vi "WPI_I2CBusCache.vi"(7 "Operation":T2, 8 "error in":errorcluster, 9 "I2C Bus":T1, 11 "Device Address":u8) -> (0 "error out":errorcluster, 2 "Allocated?":bool, 3 "Device Address Allocated":u8)   [LabVIEW 2017]
doc: "This software is licensed. Open the labview\\readme\\WPI Robotics Library Open Source License.txt file for more information."
uses:
  <vilib>/Rock Robotics/WPI/SPI/WPI_SPIBusCacheOp.ctl
  <vilib>/Rock Robotics/SystemInterfaces/i2clib/i2c_bus.ctl
  <vilib>/Rock Robotics/WPI/PWM/WPI_PWMChannelCacheOp.ctl
  <vilib>/Rock Robotics/WPI/MXP/WPI_MXP I2C Bus to first MXP Pin.vi
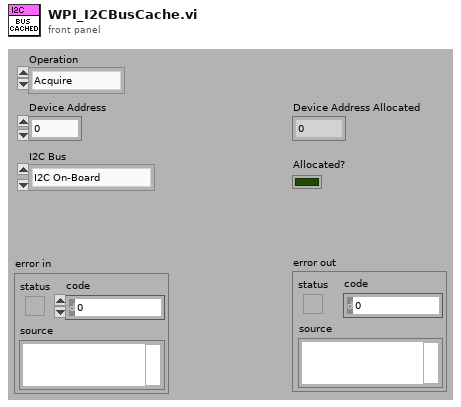
[diagram p1: front panel]
types:
  T1 = typedef "i2c_bus.ctl" = enum16{"I2C On-Board", "I2C MXP", "Invalid"}
  T2 = typedef "WPI_SPIBusCacheOp.ctl" = enum16{"Acquire", "Release", "Status"}
  T3 = typedef "WPI_PWMChannelCacheOp.ctl" = enum16{"Acquire", "Release", "Status"}
  T4 = typedef "WPI_MXP Shared MXP Pin.ctl" = enum16{"11", "13", "15", "17", "19", "21", "23", "25", "27", "29", "31", "18", "22", "26", "32", "34", "Invalid"}
  T5 = typedef "Semaphore RefNum" = refnum<k1>
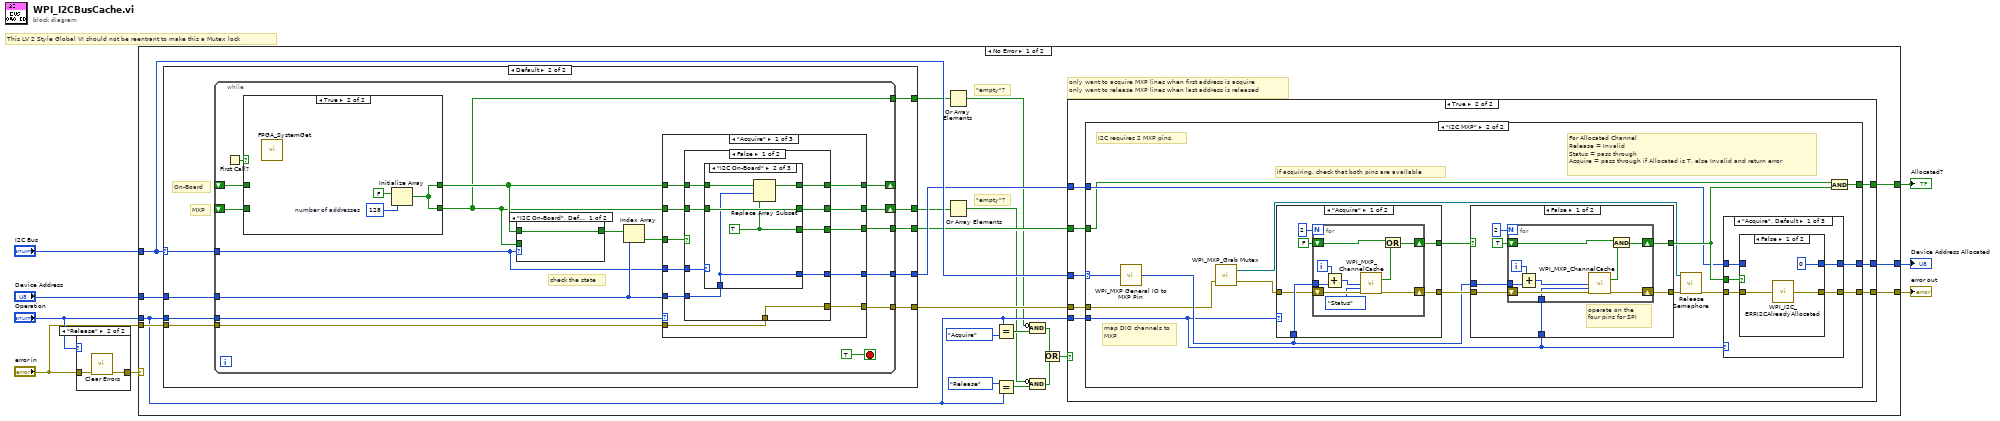
[diagram p0: block diagram]
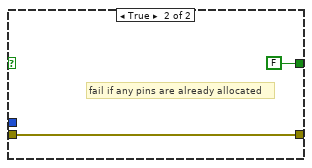
[diagram p5: hidden frame]
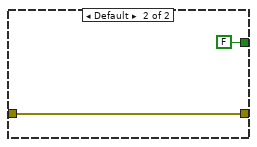
[diagram p6: hidden frame]
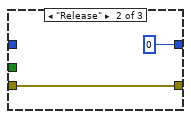
[diagram p8: hidden frame]
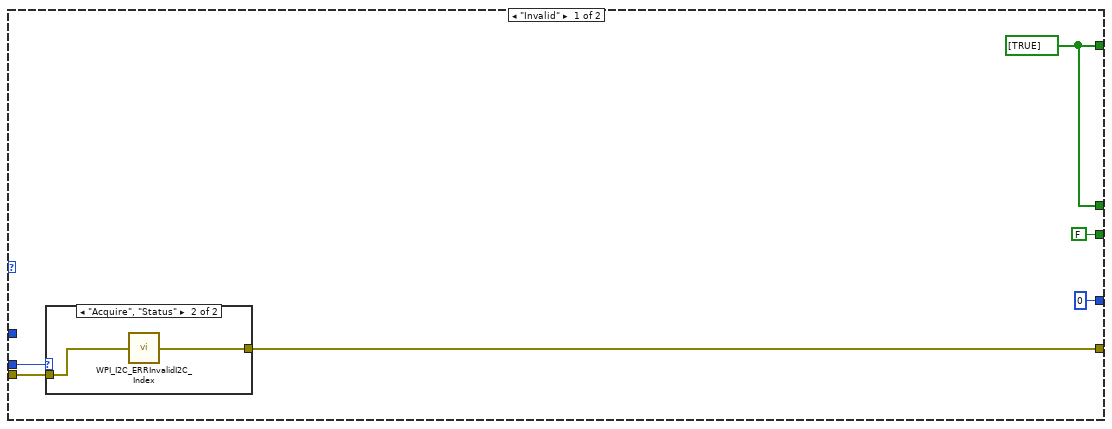
[diagram p10: hidden frame]
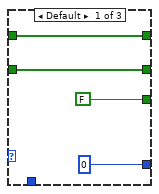
[diagram p13: hidden frame]
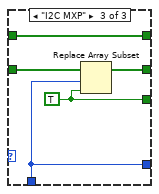
[diagram p14: hidden frame]
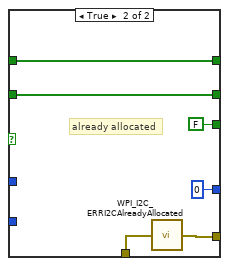
[diagram p15: hidden frame]
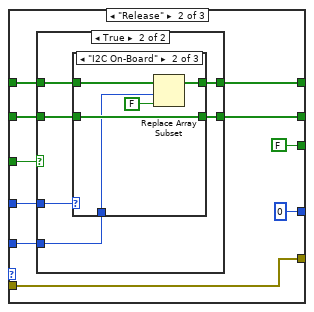
[diagram p16: hidden frame]
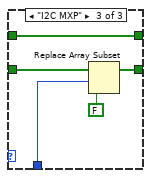
[diagram p19: hidden frame]
diagram:
  # "This LV 2 Style Global VI should not be reentrant to make this a Mutex lock"
  n1 = case shown="\"Release\"" "Operation" {
    tunnel: "error in" -> [w9 w11]
    tunnel: [w9 w10] -> w6
    frame "Acquire", Default {
    }
    frame "Release" {
      n2 = call <vilib>:"Clear Errors.vi"("error in (no error)"=w11) -> ("error out"=w10:errorcluster)  [unwired: 1 in, 5 out]
    }
  }
  n3 = case shown="No Error" w6 {
    selector: w6 -> [_ w231]
    tunnel: "Operation" -> [w19 _]
    tunnel: "Device Address" -> [w31 _]
    tunnel: [w29 w231] -> w4
    tunnel: [w30 FALSE ("new element/subarray")] -> w8
    tunnel: "I2C Bus" -> [w27 _]
    tunnel: [w26 u8 0 ("Device Address")] -> w1
    tunnel: "error in" -> [w32 _]
    frame No Error {
      # "\"empty\"?"
      # "\"empty\"?"
      # "only want to acquire MXP lines when first address is acquire\nonly want to release MXP lines when last address is released"
      n4 = case shown="Default" w27 {
        selector: w27 -> [_ w123]
        tunnel: w19 -> [w117 w129]
        tunnel: [w116 w128] -> w28
        tunnel: [FALSE ("new element/subarray") w127] -> w24
        tunnel: [u8 0 ("Device Address Allocated") w126] -> w25
        tunnel: w32 -> [w115 w125]
        tunnel: w31 -> [_ w124]
        tunnel: [w112 w122] -> w23
        tunnel: [w112 w121] -> w16
        frame "Invalid" {
          w112 = bool[] [TRUE]
          n5 = case shown="\"Acquire\", \"Status\"" w117 {
            tunnel: [w118 w120] -> w116
            tunnel: w115 -> [w118 w119]
            frame "Release" {
            }
            frame "Acquire", "Status" {
              n6 = call <vilib>:"WPI_I2C_ERRInvalidI2C_Index.vi"("error in (no error)"=w119) -> ("error out"=w120:errorcluster)
            }
          }
        }
        frame Default {
          # "MXP"
          # "On-Board"
          n7 = while {
            shift-right: [w143] -> _
            shift-left: _ -> [w145]
            tunnel: w129 -> [w144]
            tunnel: w124 -> [w137]
            tunnel: [w142] -> w128
            tunnel: [w141] -> w127
            shift-right: [w139] -> w121
            shift-left: _ -> [w140]
            tunnel: w123 -> [w133]
            tunnel: [w136] -> w126
            tunnel: w125 -> [w134]
            tunnel: [w132] -> w122
            stop <- TRUE stop-if-true
            # "check the state"
            n8 = First Call?() -> (First Call?: T/F=w146:bool)
            n9 = case shown="True" w146 {
              tunnel: w145 -> [w225 _]
              tunnel: [w225 w228] -> w138
              tunnel: [w224 w228] -> w132
              tunnel: w140 -> [w224 _]
              frame False {
              }
              frame True {
                w227 = 128  # number of addresses
                n10 = call <vilib>:"FPGA_SystemGet.vi"() -> ()  [unwired: 11 in, 1 out]
                n11 = Initialize Array(FALSE, w227) -> (w228:bool[])
              }
            }
            n12 = case shown="\"I2C On-Board\", Default" w133 {
              tunnel: w138 -> [w147 _]
              tunnel: [w147 w148] -> w131
              tunnel: w132 -> [_ w148]
              frame "I2C On-Board", Default {
              }
              frame "I2C MXP" {
              }
            }
            n13 = Index Array(array=w131, index=w137) -> (element=w130:bool)
            n14 = case shown="\"Acquire\"" w144 {
              tunnel: w138 -> [w155 w198 w222]
              tunnel: [w159 w196 w222] -> w143
              tunnel: w137 -> [w158 w197 w220]
              tunnel: [w157 w191 w219] -> w142
              tunnel: [w156 FALSE ("new element/subarray") w221] -> w141
              tunnel: w132 -> [w154 w194 w223]
              tunnel: [w150 w193 w223] -> w139
              tunnel: w130 -> [w153 w195 w221]
              tunnel: w133 -> [w152 w192 _]
              tunnel: [w151 u8 0 ("Device Address") w220] -> w136
              tunnel: w134 -> [w149 w191 w219]
              frame "Acquire" {
                n15 = case shown="False" w153 {
                  tunnel: w155 -> [w165 w188]
                  tunnel: [w164 w188] -> w159
                  tunnel: w158 -> [w168 _]
                  tunnel: [w160 w186] -> w157
                  tunnel: [w167 FALSE ("new element/subarray")] -> w156
                  tunnel: w154 -> [w163 w187]
                  tunnel: [w162 w187] -> w150
                  tunnel: w152 -> [w166 _]
                  tunnel: [w161 u8 0 ("Device Address Allocated")] -> w151
                  tunnel: w149 -> [w160 w185]
                  frame False {
                    n16 = case shown="\"I2C On-Board\"" w166 {
                      tunnel: w168 -> [_ w174 w179]
                      tunnel: [FALSE ("new element/subarray") w173 w178] -> w167
                      tunnel: w165 -> [w172 w176 w182]
                      tunnel: [w172 w175 w182] -> w164
                      tunnel: w163 -> [w171 w177 w181]
                      tunnel: [w171 w177 w180] -> w162
                      tunnel: [u8 0 ("Device Address") w174 w179] -> w161
                      frame Default {
                      }
                      frame "I2C On-Board" {
                        w173 = TRUE ("new element/subarray")
                        n17 = Replace Array Subset(array=w176, new element=w173, index=w174) -> (w175:bool[])
                      }
                      frame "I2C MXP" {
                        w178 = TRUE ("new element/subarray")
                        n18 = Replace Array Subset(array=w181, new element=w178, index=w179) -> (w180:bool[])
                      }
                    }
                  }
                  frame True {
                    # "already allocated"
                    n19 = call <vilib>:"WPI_I2C_ERRI2CAlreadyAllocated.vi"("error in (no error)"=w185) -> ("error out"=w186:errorcluster)
                  }
                }
              }
              frame "Release" {
                n20 = case shown="True" w195 {
                  tunnel: w198 -> [w200 w206]
                  tunnel: w197 -> [_ w205]
                  tunnel: [w200 w204] -> w196
                  tunnel: w194 -> [w199 w202]
                  tunnel: [w199 w201] -> w193
                  tunnel: w192 -> [_ w203]
                  frame False {
                  }
                  frame True {
                    n21 = case shown="\"I2C On-Board\"" w203 {
                      tunnel: w206 -> [w208 w212 w218]
                      tunnel: w205 -> [_ w210 w215]
                      tunnel: [w208 w211 w218] -> w204
                      tunnel: w202 -> [w207 w213 w217]
                      tunnel: [w207 w213 w216] -> w201
                      frame Default {
                      }
                      frame "I2C On-Board" {
                        n22 = Replace Array Subset(array=w212, new element=FALSE ("new element/subarray"), index=w210) -> (w211:bool[])
                      }
                      frame "I2C MXP" {
                        n23 = Replace Array Subset(array=w217, new element=FALSE ("new element/subarray"), index=w215) -> (w216:bool[])
                      }
                    }
                  }
                }
              }
              frame "Status" {
              }
            }
          }
        }
      }
      n24 = Or Array Elements(Boolean array=w23) -> (logical OR=w14:bool)
      n25 = Or Array Elements(Boolean array=w16) -> (logical OR=w13:bool)
      n26 = Equal?(x=w19, y=WPI_SPIBusCacheOp."Acquire" ("Operation")) -> (x = y?=w21:bool)
      n27 = Equal?(x=WPI_SPIBusCacheOp."Release" ("Operation"), y=w19) -> (x = y?=w15:bool)
      n28 = Compound Arithmetic op=AND(invert w14, w21) -> (w17:bool)
      n29 = Compound Arithmetic op=AND(invert w13, w15) -> (w12:bool)
      n30 = Or(x=w17, y=w12) -> (x .or. y?=w18:bool)
      n31 = case shown="True" w18 {
        tunnel: [w35 w43] -> w30
        tunnel: [w33 w42] -> w29
        tunnel: w28 -> [w33 w41]
        tunnel: w27 -> [_ w40]
        tunnel: w19 -> [_ w39]
        tunnel: [w34 w38] -> w26
        tunnel: w25 -> [w34 w37]
        tunnel: w24 -> [w35 w36]
        frame False {
        }
        frame True {
          n32 = case shown="\"I2C MXP\"" w40 {
            selector: w40 -> [_ w60]
            tunnel: w39 -> [_ w56]
            tunnel: [w46 w62] -> w42
            tunnel: [w44 w48] -> w43
            tunnel: [w45 w61] -> w38
            tunnel: w41 -> [w46 w52]
            tunnel: w37 -> [w45 w49]
            tunnel: w36 -> [w44 w47]
            frame Default {
            }
            frame "I2C MXP" {
              # "I2C requires 2 MXP pins."
              # "if acquiring, check that both pins are available"
              # "map DIO channels to MXP"
              # "For Allocated Channel\nRelease = Invalid\nStatus = pass through\nAcquire = pass through if Allocated is T, else Invalid and return error"
              n33 = call-poly <vilib>:"WPI_MXP General IO to MXP Pin.vi"("I2C Bus"=w60) -> ("Shared MXP Pin"=w57:T4)  [unwired: 14 in]
              n34 = call <vilib>:"WPI_MXP_Grab Mutex.vi"("error in"=w52) -> ("error out"=w51:errorcluster, "semaphore out"=w50:T5)  [unwired: 1 in]
              n35 = case shown="\"Acquire\"" w56 {
                tunnel: [w86 w97] -> w59
                tunnel: w57 -> [w85 _]
                tunnel: w51 -> [w84 w97]
                tunnel: [w81 FALSE] -> w58
                frame "Acquire" {
                  n36 = for {
                    N: 2 -> [_]
                    tunnel: w85 -> [w94]
                    shift-right: [w95] -> w86
                    shift-left: w84 -> [w93]
                    shift-right: [w90] -> w81
                    shift-left: FALSE -> [w89]
                    i -> [w91]
                    n37 = Add(x=w91, y=w94) -> (x+y=w92:i32)
                    n38 = call <vilib>:"WPI_MXP_ChannelCache.vi"("Shared MXP Pin"=w92, "Operation"=WPI_PWMChannelCacheOp."Status", "error in (no error)"=w93) -> ("Allocated?"=w88:bool, "error out"=w95:errorcluster)  [unwired: 11 in]
                    n39 = Or(x=w89, y=w88) -> (x .or. y?=w90:bool)
                  }
                }
                frame Default {
                }
              }
              n40 = case shown="False" w58 {
                tunnel: [w69 w80] -> w54
                tunnel: w57 -> [w68 _]
                tunnel: w59 -> [w67 w80]
                tunnel: [w64 FALSE] -> w55
                tunnel: w56 -> [w63 _]
                frame False {
                  # "operate on the four pins for SPI"
                  n41 = for {
                    N: 2 -> [_]
                    tunnel: w68 -> [w77]
                    shift-right: [w78] -> w69
                    shift-left: w67 -> [w76]
                    shift-right: [w73] -> w64
                    shift-left: TRUE -> [w72]
                    tunnel: w63 -> [w70]
                    i -> [w74]
                    n42 = Add(x=w74, y=w77) -> (x+y=w75:i32)
                    n43 = call <vilib>:"WPI_MXP_ChannelCache.vi"("Shared MXP Pin"=w75, "Operation"=w70, "error in (no error)"=w76) -> ("Allocated?"=w71:bool, "error out"=w78:errorcluster)  [unwired: 11 in]
                    n44 = And(x=w72, y=w71) -> (x .and. y?=w73:bool)
                  }
                }
                frame True {
                  # "fail if any pins are already allocated"
                }
              }
              n45 = call <vilib>:"Release Semaphore.vi"("error in (no error)"=w54, "semaphore"=w50) -> ("error out"=w53:errorcluster)  [unwired: 4 in, 1 out]
              n46 = case shown="\"Acquire\", Default" w56 {
                tunnel: [w101 u8 0 ("Device Address Allocated") w111] -> w61
                tunnel: w49 -> [w100 _ w111]
                tunnel: w53 -> [w99 w109 w110]
                tunnel: w55 -> [w102 _ _]
                tunnel: [w98 w109 w110] -> w62
                frame "Acquire", Default {
                  n47 = case shown="False" w102 {
                    tunnel: [u8 0 ("Device Address Allocated") w107] -> w101
                    tunnel: w100 -> [_ w107]
                    tunnel: w99 -> [w104 w106]
                    tunnel: [w105 w106] -> w98
                    frame False {
                      n48 = call <vilib>:"WPI_I2C_ERRI2CAlreadyAllocated.vi"("error in (no error)"=w104) -> ("error out"=w105:errorcluster)
                    }
                    frame True {
                    }
                  }
                }
                frame "Release" {
                }
                frame "Status" {
                }
              }
              n49 = And(x=w47, y=w55) -> (x .and. y?=w48:bool)
            }
          }
        }
      }
    }
    frame Error {
    }
  }
  "Allocated?" <- w8
  "error out" <- w4
  "Device Address Allocated" <- w1
